vi "XPARTD_ExecParams.vi"(7 "display":string, 8 "error in (no error)":errorcluster, 10 "params in":string[](array[string]), 11 "xpapath":string) -> (0 "error out":errorcluster, 2 "resp":string[](array[string]))   [LabVIEW 2016]
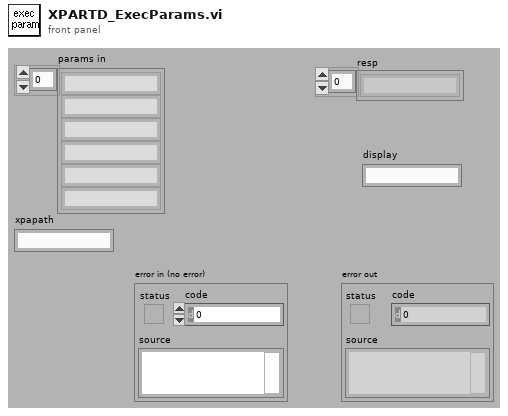
[diagram p1: front panel]
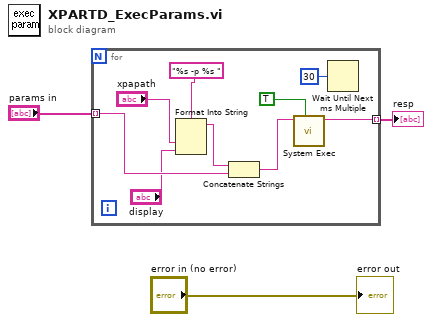
[diagram p0: block diagram]
diagram:
  n1 = for {
    tunnel: "params in" -> [w8] mode=indexing
    tunnel: [w4] -> w1 mode=indexing
    n2 = Format Into String(format string="%s -p %s ", "xpapath", "display") -> (resulting string=w9:string)  [unwired: 2 in, 1 out]
    n3 = Concatenate Strings(w9, w8) -> (w7:string)
    n4 = call <vilib>:"System Exec.vi"("wait until completion? (T)"=TRUE, "command line"=w7) -> ("standard output"=w4:string)  [unwired: 4 in, 5 out]
    n5 = Wait Until Next ms Multiple(millisecond multiple=u32 30) -> ()  [unwired: 1 out]
  }
  "resp" <- w1
  "error out" <- "error in (no error)"
